vi "ring command from db.vi"(8 "error in":errorcluster, 11 "IOC":string) -> (0 "error out":errorcluster, 3 "Strings And Values Commands":cluster{"String":string, "Value":string}[](array[cluster]))   [LabVIEW 2022 SP3]
uses:
  pectus/global/global IOC database.vi
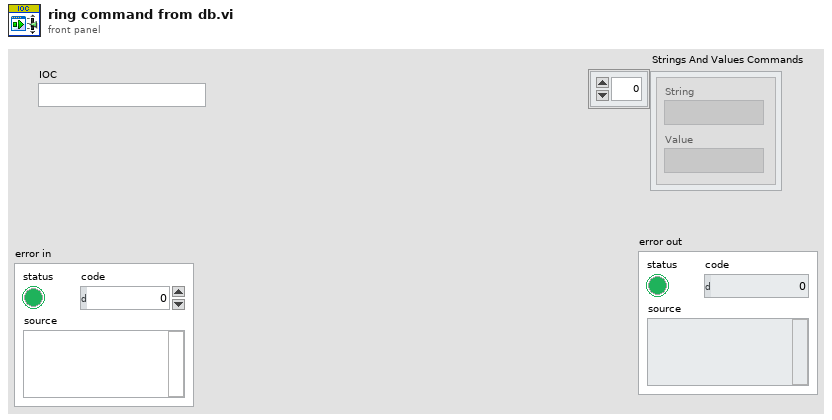
[diagram p1: front panel]
types:
  T1 = typedef "epics database.ctl" = cluster{"IOC":string, "db":string, "Field Values":string[], "Values":string[][], "Type":string, "Card":u16, "Num Dev":u16}
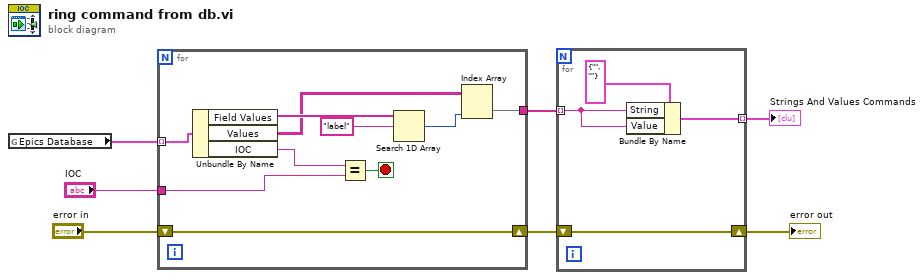
[diagram p0: block diagram]
diagram:
  n1 = global read "global IOC database.vi" "Epics Database"() -> (w7:T1[])
  n2 = for {
    tunnel: w7 -> [w17] mode=indexing
    tunnel: "IOC" -> [w15]
    shift-right: [w10] -> w4
    shift-left: "error in" -> [w10]
    tunnel: [w9] -> w2
    stop <- w8 stop-if-true
    n3 = Unbundle By Name(w17) -> ("Field Values"=w14:string[], "Values"=w12:string[][], "IOC"=w16:string)
    n4 = Equal?(x=w16, y=w15) -> (x = y?=w8:bool)
    n5 = Search 1D Array(1D array=w14, element="label") -> (index of element=w11:i32)  [unwired: 1 in]
    n6 = Index Array(array=w12, index (col)=w11) -> (element=w9:string[])  [unwired: 1 in]
  }
  n7 = for {
    shift-right: [w21] -> w3
    shift-left: w4 -> [w21]
    tunnel: w2 -> [w19] mode=indexing
    tunnel: [w18] -> w1 mode=indexing
    n8 = Bundle By Name(cluster=cluster{"String":string, "Value":string} {"String"="", "Value"=""}, "String"=w19, "Value"=w19) -> (w18:cluster{"String":string, "Value":string})
  }
  "error out" <- w3
  "Strings And Values Commands" <- w1
